vi "Task B.vi"(8 "error in (no error)":errorcluster caption="错误输入（无错误）") -> (0 "error out":errorcluster caption="错误输出")   [LabVIEW 2013]
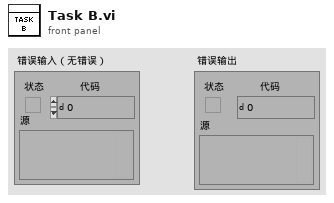
[diagram p1: front panel]
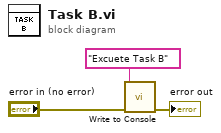
[diagram p0: block diagram]
diagram:
  n1 = call "Write to Console.vi"("error in (no error)"="error in (no error)", "Input"="Excuete Task B") -> ("error out"=→"error out":errorcluster)  [unwired: 9 in]
